vi "_014.vi"() -> ()   [LabVIEW 2024]
uses:
  <vilib>/Utility/error.llb/whitespace.ctl
  <vilib>/Utility/error.llb/Trim Whitespace One-Sided.vi
panel:
  in  "location (both)":T1 items=["both", "start of string", "end of string"]
  out "trimmed string":string
  in  "string 4":string
  out "substring":string
  in  "length (rest)":i32
  in  "offset (0)":i32
  in  "string":string
  in  "string 2":string
  out "concatenated string":string
  in  "string 1":string
  out "length":i32
  in  "string":string
  # "String functions :"
  # "(Basics)"
  # "String Length :"
  # "Concordinate Strings :"
  # "String Subset :"
  # "Trim Whitespace :"
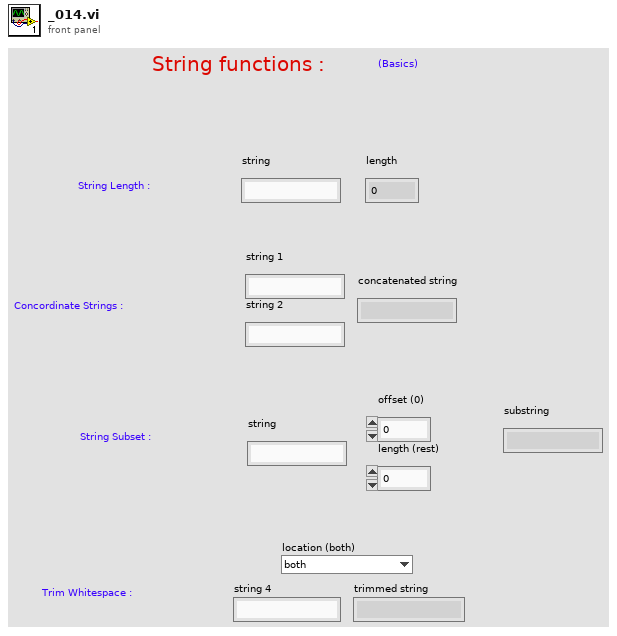
[diagram p1: front panel]
types:
  T1 = typedef "whitespace.ctl" = u16
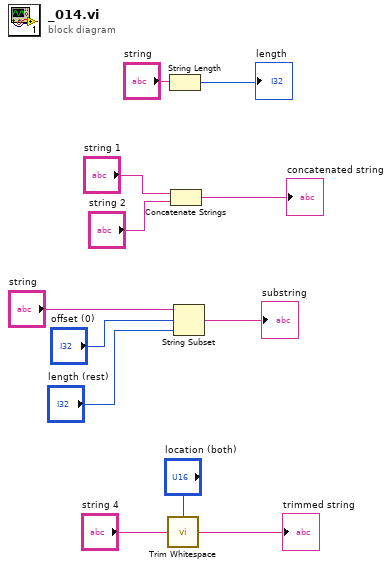
[diagram p0: block diagram]
diagram:
  n1 = call <vilib>:"Trim Whitespace.vi"("string"="string 4", "location (both)"="location (both)") -> ("trimmed string"=→"trimmed string":string)
  n2 = String Length(string="string") -> (length=→"length":i32)
  n3 = Concatenate Strings "Concatenate Strings"("string 1", "string 2") -> (→"concatenated string":string)
  n4 = String Subset(string="string", offset (0)="offset (0)", length (rest)="length (rest)") -> (substring=→"substring":string)
